vi "Set Ref plots img window UI from file.vi"(8 "error in (no error)":errorcluster, 9 "Keys setup.DBL":T2, 10 "Section name":string, 11 "Refnum in":T1) -> (0 "error out":errorcluster, 3 "Refnum out":T1)   [LabVIEW 2020]
uses:
  Typedefs/Ini file interface (DBL).ctl
  <vilib>/Utility/config.llb/Config Data RefNum.ctl
  User Interface/Globals/gl_Windows Ctrl refs.vi
  <vilib>/Utility/config.llb/NI_LVConfig.lvlib
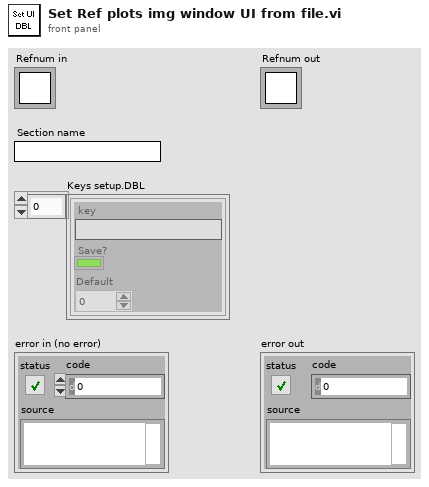
[diagram p1: front panel]
types:
  T1 = typedef "NI_LVConfig.lvlib/Config Data RefNum.ctl" = refnum<k1>
  T2 = typedef "Ini file interface (DBL).ctl" = cluster{"key":string, "Save?":bool, "Default":dbl}[]
  T3 = typedef "Reference plots window ctrl refs.ctl" = cluster{"Refresh rate (ms)":refnum<vi>, "Buffer Size":refnum<vi>}
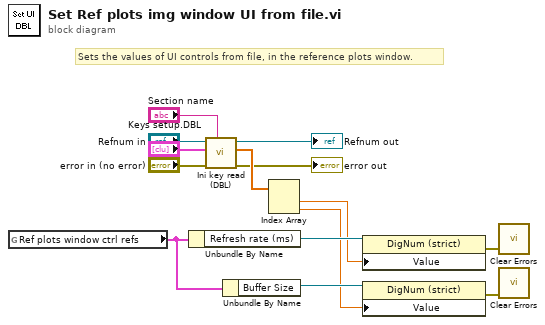
[diagram p0: block diagram]
diagram:
  # "Sets the values of UI controls from file, in the reference plots window."
  n1 = global read "gl_Windows Ctrl refs.vi" "Ref plots window ctrl refs"() -> (w6:T3)
  n2 = Unbundle By Name(w6) -> ("Refresh rate (ms)"=w5:refnum<vi>)
  n3 = call "Ini key read (DBL).vi"("Section name"="Section name", "error in (no error)"="error in (no error)", "Parameter names & setup"="Keys setup.DBL", "Ini file refnum in"="Refnum in") -> ("error out"=→"error out":errorcluster, "Value read/used"=w12:dbl[], "Ini file refnum out"=→"Refnum out":T1)  [unwired: 5 in]
  n4 = Unbundle By Name(w6) -> ("Buffer Size"=w4:refnum<vi>)
  n5 = Index Array(array=w12) -> (element #1=w3:dbl, element #2=w2:dbl)  [unwired: 2 in]
  n6 = property class="DigNum (strict)"(reference=w5, "Value"=w3) -> (error out=w1:errorcluster)  [unwired: 1 in, 1 out]
  n7 = property class="DigNum (strict)"(reference=w4, "Value"=w2) -> (error out=w7:errorcluster)  [unwired: 1 in, 1 out]
  n8 = call <vilib>:"Clear Errors.vi"("error in (no error)"=w1) -> ()  [unwired: 5 in, 2 out]
  n9 = call <vilib>:"Clear Errors.vi"("error in (no error)"=w7) -> ()  [unwired: 5 in, 2 out]
